vi "Sort.vi"() -> ()   [LabVIEW 2012]
uses:
  <vilib>/Analysis/1siggen.llb/Riffle Array (I32).vi
  <vilib>/Analysis/NI_AALBase.lvlib
panel:
  out "current time":timestamp
  out "Last Max Index":i32
  in  "Reset":bool
  in  "Sort Type:":u16(ring) items=["Labview Sort", "Bubble", "Insertion", "Selection"]
  out "Sort array":i32[](array[numeric])
  in  "EXIT":bool
  in  "GO":bool
  out "Raw Data":waveform(i32)(graph)
  # "There is a 20ms delay in sort loops so that the sorts happen slow enough to veiw.\nThis affects the \"Time took to sort\". Also the sample size is 100 non-recurring numbers from 1-100."
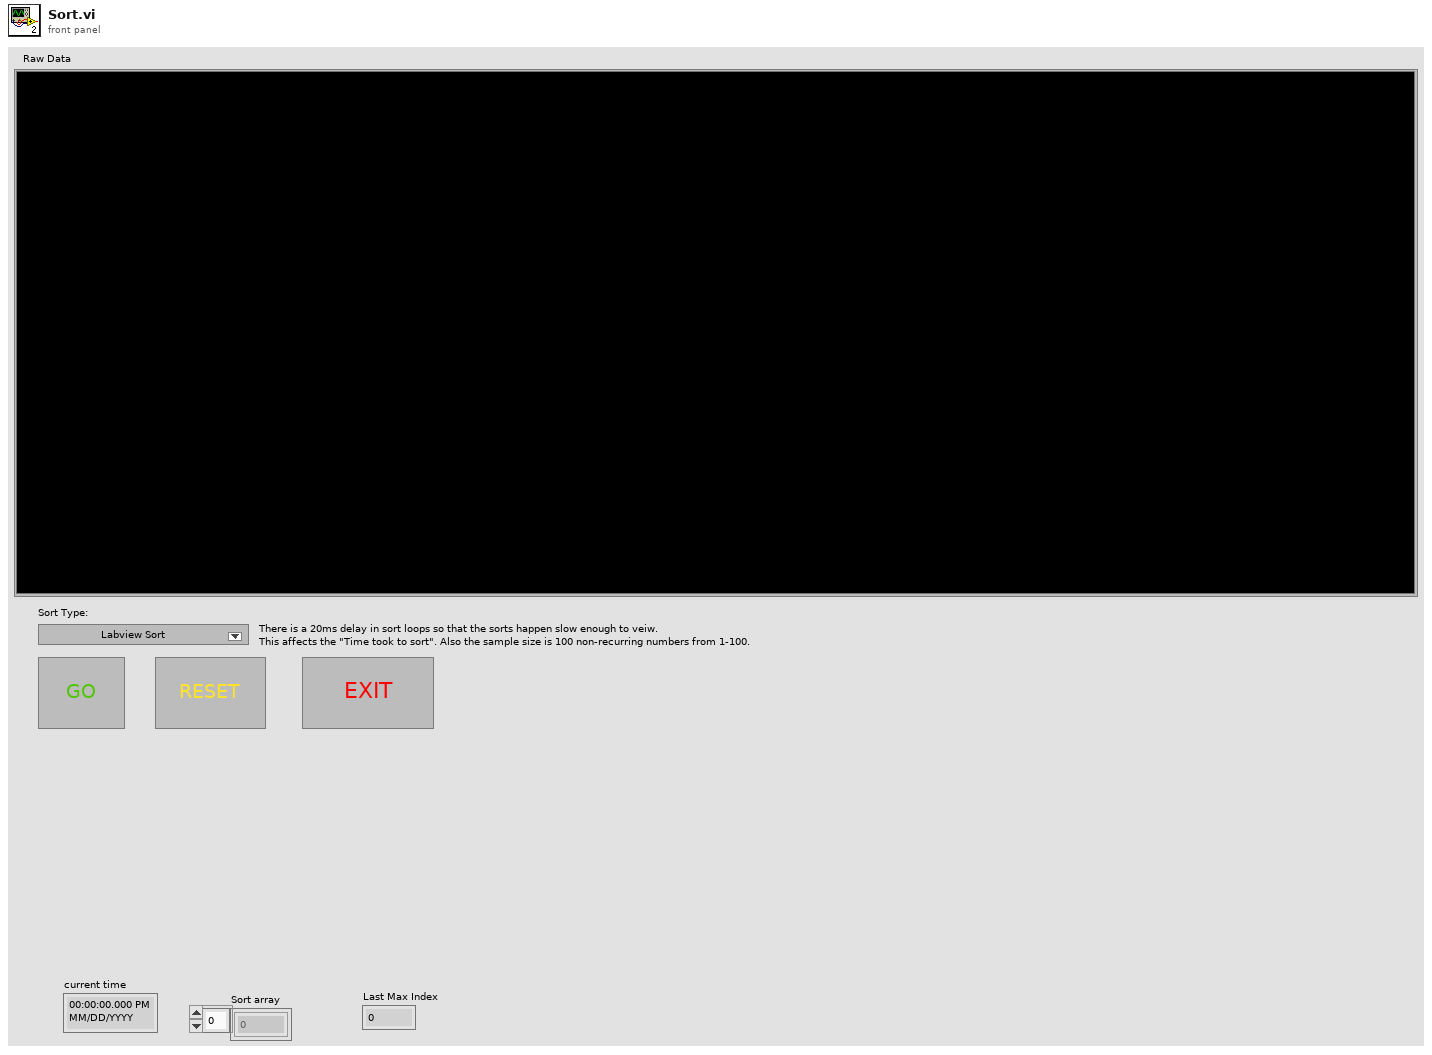
[diagram p1: front panel]
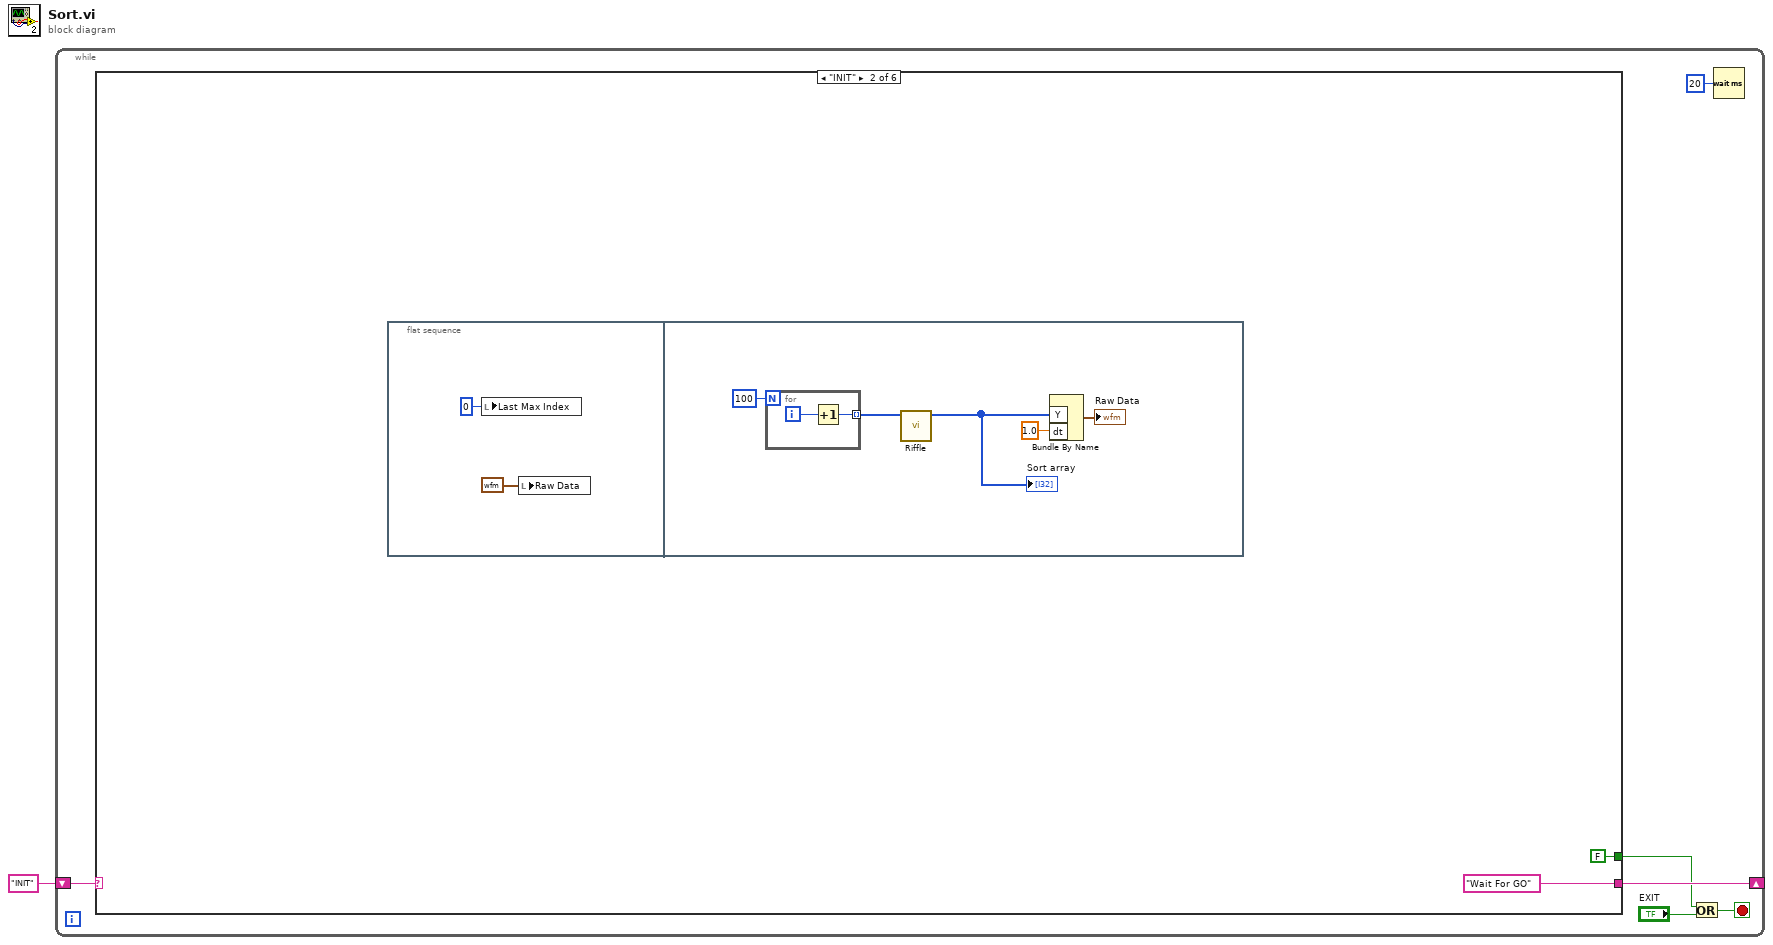
[diagram p0: block diagram]
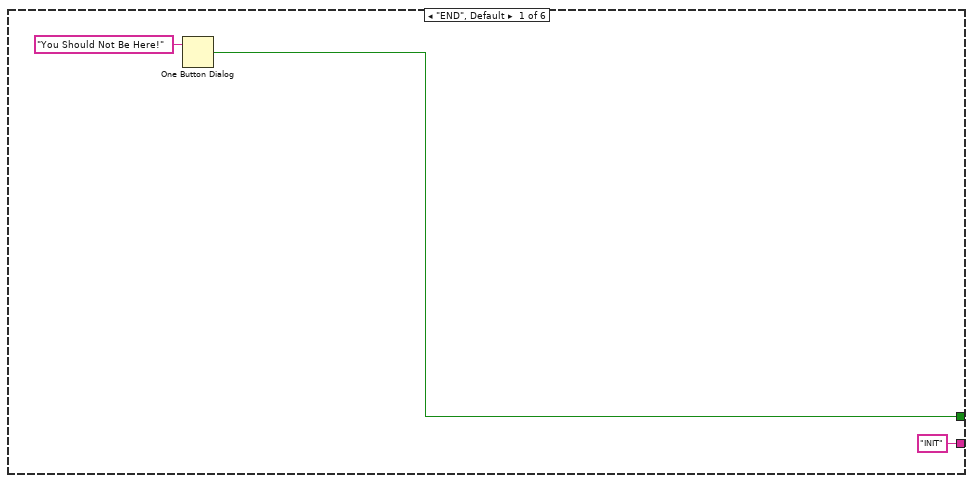
[diagram p2: hidden frame]
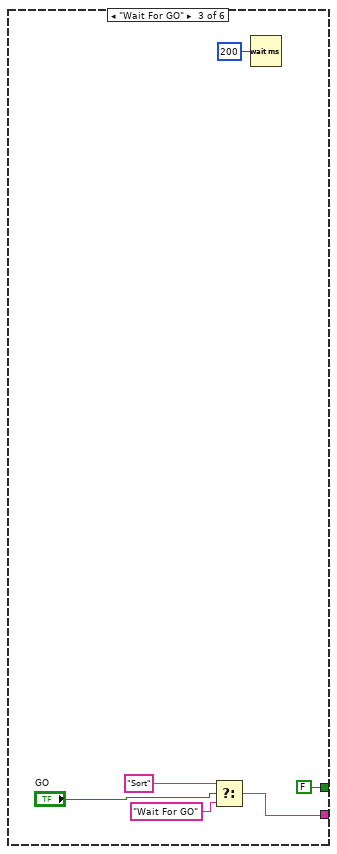
[diagram p3: hidden frame]
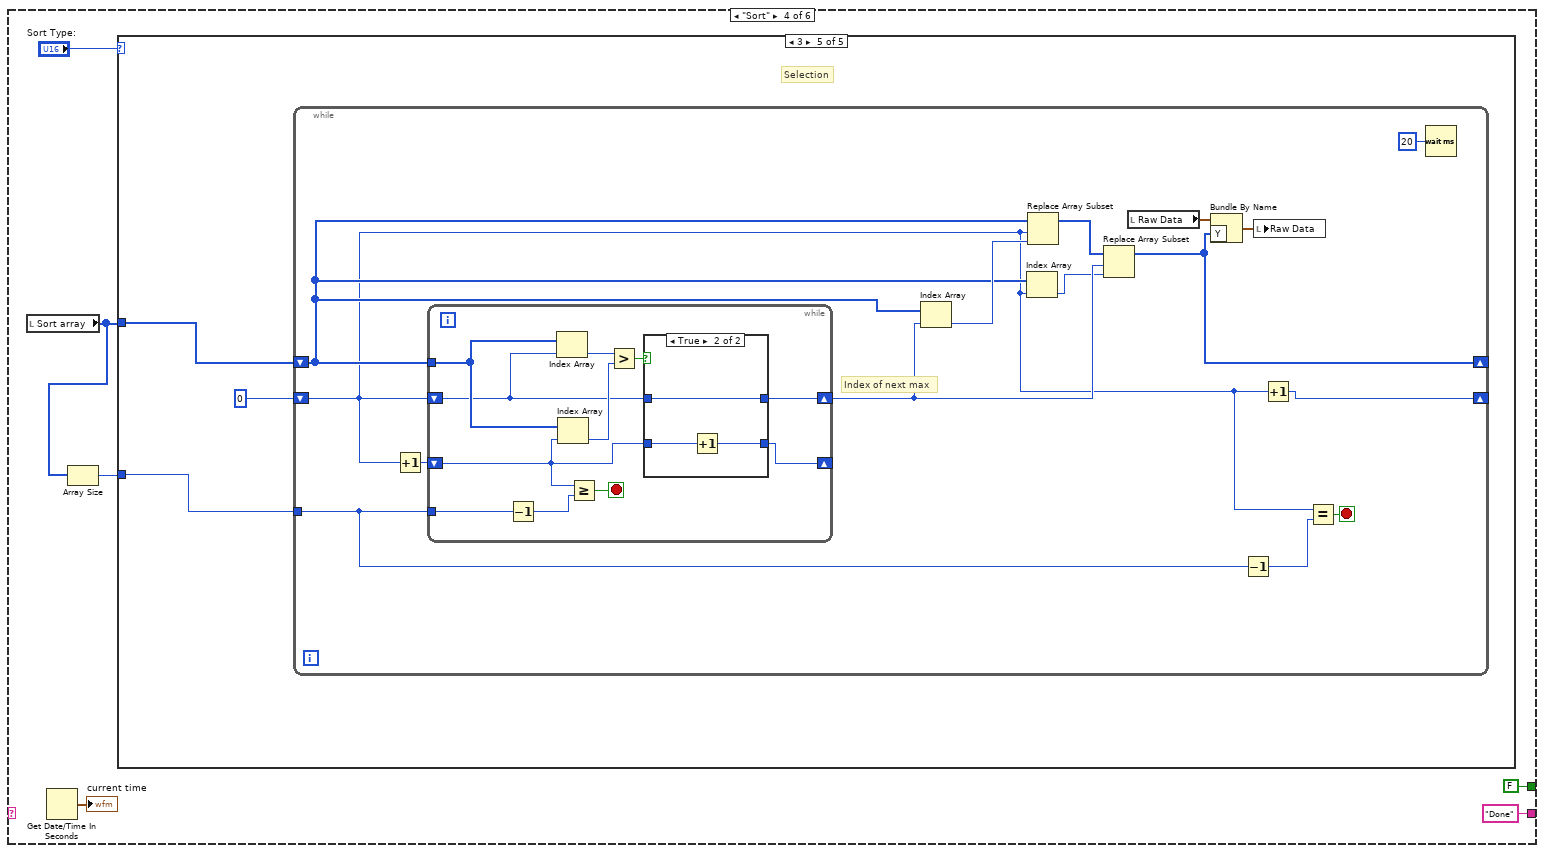
[diagram p4: hidden frame]
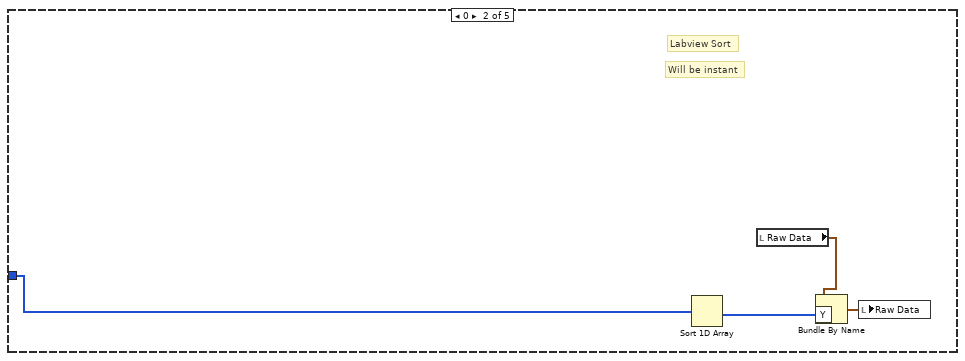
[diagram p6: hidden frame]
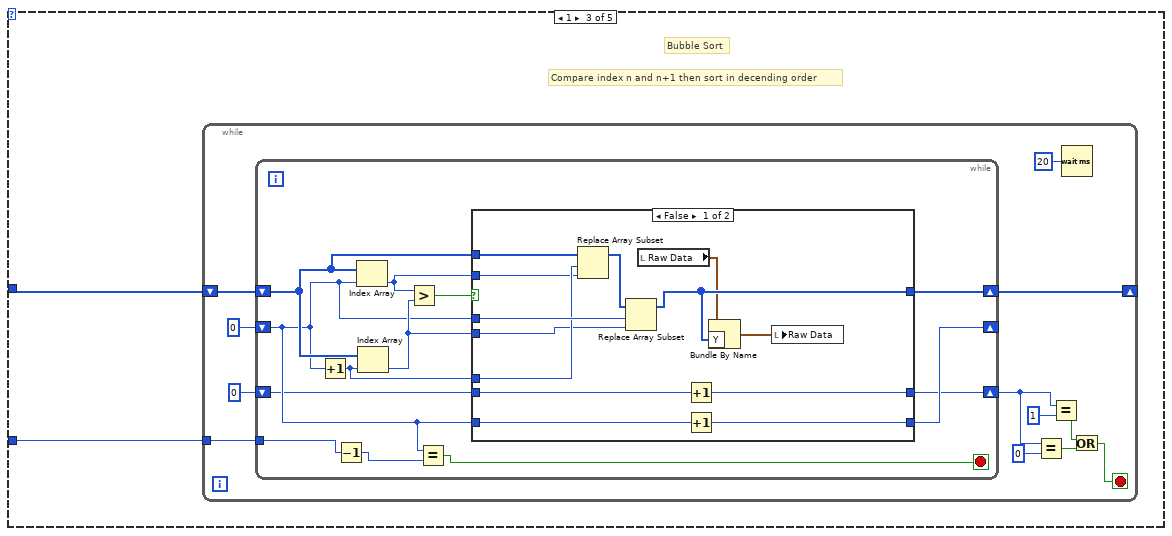
[diagram p7: hidden frame]
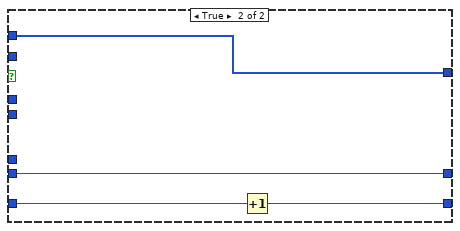
[diagram p8: hidden frame]
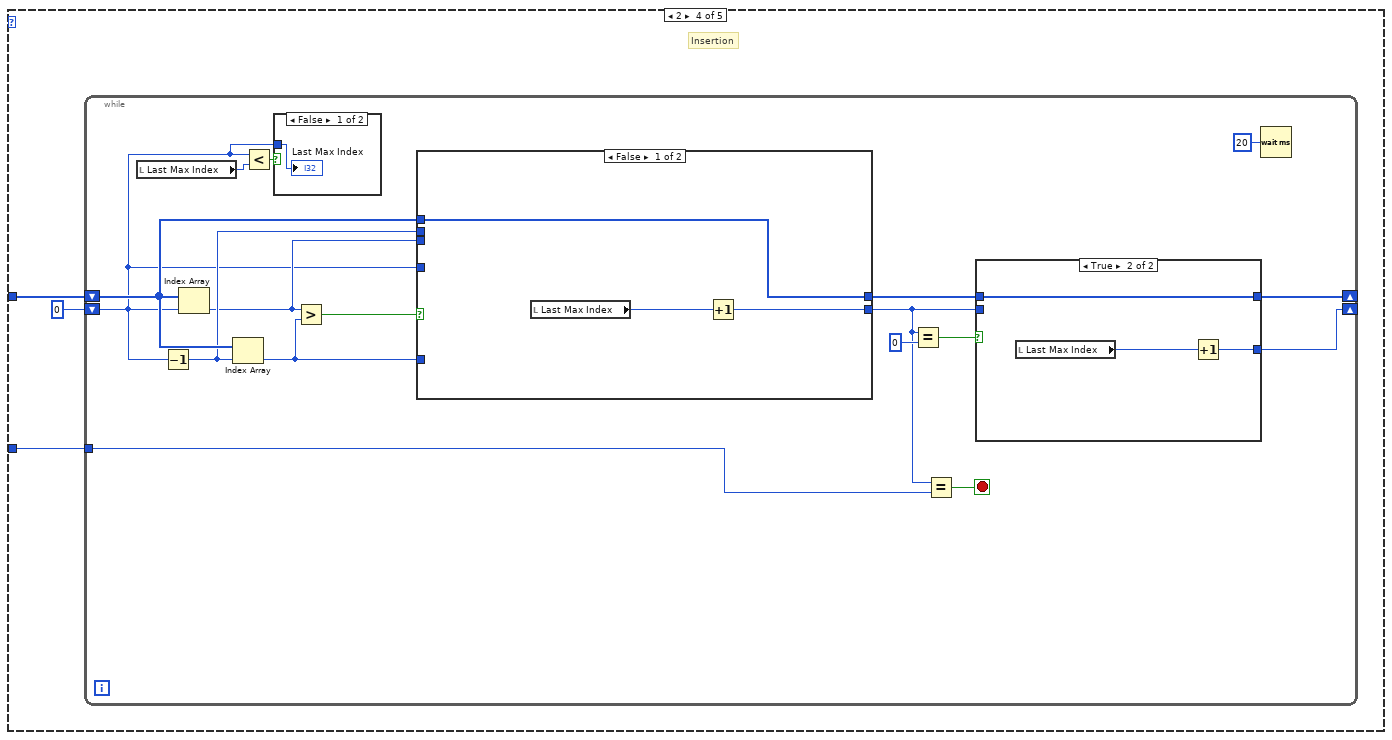
[diagram p9: hidden frame]
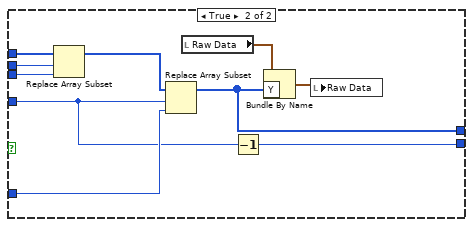
[diagram p12: hidden frame]
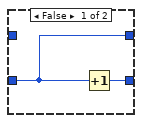
[diagram p13: hidden frame]
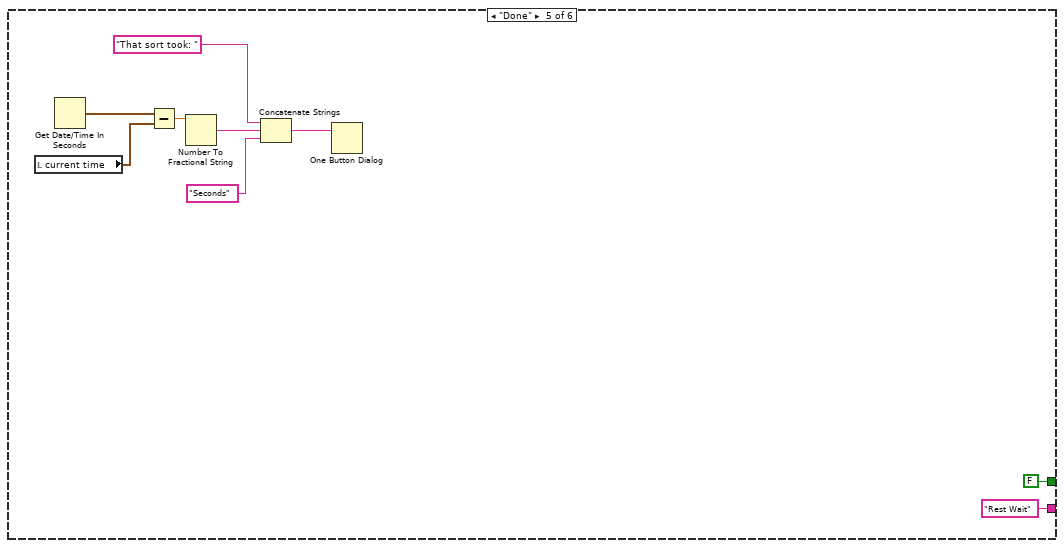
[diagram p14: hidden frame]
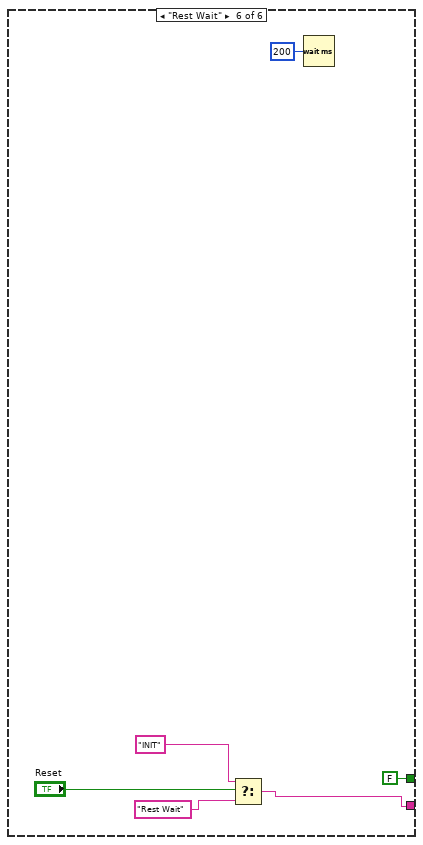
[diagram p15: hidden frame]
diagram:
  n1 = while {
    shift-right: [w5] -> _
    shift-left: "INIT" -> [w6]
    stop <- w4 stop-if-true
    n2 = case shown="\"INIT\"" w6 {
      tunnel: ["INIT" ("f") "Wait For GO" ("f") w23 "Done" ("f") "Rest Wait" ("f") w168] -> w5
      tunnel: [w9 FALSE ("true") FALSE ("true") FALSE ("true") FALSE ("true") FALSE ("true")] -> w2
      frame "END", Default {
        n3 = One Button Dialog(message="You Should Not Be Here!") -> (true=w9:bool)  [unwired: 1 in]
      }
      frame "INIT" {
        n4 = flat-sequence {
          frame #0 {
            n5 = local write "Last Max Index"(0 ("Last Max Index")) -> ()
            n6 = local write "Raw Data"(waveform(dbl) {"t0"=timestamp(0 s since 1904-01-01), "dt"=0.0, "Y"=[]} ("output waveform")) -> ()
          }
          frame #1 {
            n7 = for {
              N: 100 -> [_]
              tunnel: [w20] -> w16 mode=indexing
              i -> [w21]
              n8 = Increment(x=w21) -> (x+1=w20:i32)
            }
            n9 = call-poly <vilib>:"Riffle.vi"("X"=w16) -> ("Riffled {X}"=w15:i32[])  [unwired: 8 in, 2 out]
            "Sort array" <- w15
            n10 = Bundle By Name("Y"=w15, "dt"=1.0) -> (→"Raw Data":waveform(i32))  [unwired: 1 in]
          }
        }
      }
      frame "Wait For GO" {
        n11 = Select(t="Sort", s="GO", f="Wait For GO") -> (s? t:f=w23:string)
        n12 = Wait (ms)(milliseconds to wait=u32 200) -> ()  [unwired: 1 out]
      }
      frame "Sort" {
        n13 = local read "Sort array"() -> (w31:i32[])
        n14 = Get Date/Time In Seconds() -> (seconds since 1Jan1904=→"current time":timestamp)
        n15 = Array Size(array=w31) -> (size(s)=w32:i32)
        n16 = case shown="3" "Sort Type:" {
          tunnel: w32 -> [_ _ w39 w82 w122]
          tunnel: w31 -> [_ w37 w38 w84 w123]
          frame Default {
          }
          frame 0 {
            # "Will be instant"
            # "Labview Sort"
            n17 = Sort 1D Array(array=w37) -> (sorted array=w34:i32[])
            n18 = local read "Raw Data"() -> (w35:waveform(i32))
            n19 = Bundle By Name(cluster=w35, "Y"=w34) -> (w36:waveform(i32))
            n20 = local write "Raw Data"(w36) -> ()
          }
          frame 1 {
            # "Compare index n and n+1 then sort in decending order"
            # "Bubble Sort"
            n21 = while {
              tunnel: w39 -> [w49]
              shift-right: [w48] -> _
              shift-left: w38 -> [w50]
              stop <- w41 stop-if-true
              n22 = while {
                shift-right: [w59] -> w48
                shift-left: w50 -> [w63]
                shift-right: [w58] -> _
                shift-left: 0 ("index (row)") -> [w57]
                tunnel: w49 -> [w56]
                shift-right: [w52] -> w45
                shift-left: 0 ("index (row)") -> [w53]
                stop <- w54 stop-if-true
                n23 = Increment(x=w57) -> (x+1=w62:i32)
                n24 = Decrement(x=w56) -> (x-1=w55:i32)
                n25 = Index Array(array=w63, index=w57) -> (element=w60:i32)
                n26 = Index Array(array=w63, index=w62) -> (element=w61:i32)
                n27 = Greater?(x=w60, y=w61) -> (0:w64:bool)
                n28 = Equal?(x=w57, y=w55) -> (x = y?=w54:bool)
                n29 = case shown="False" w64 {
                  tunnel: w63 -> [w77 w79]
                  tunnel: w57 -> [w76 _]
                  tunnel: w62 -> [w75 _]
                  tunnel: w61 -> [w74 _]
                  tunnel: w60 -> [w73 _]
                  tunnel: [w70 w79] -> w59
                  tunnel: w57 -> [w71 w81]
                  tunnel: [w68 w80] -> w58
                  tunnel: w53 -> [w67 w78]
                  tunnel: [w66 w78] -> w52
                  frame False {
                    n30 = Replace Array Subset(array=w77, new element=w73, index=w75) -> (w72:i32[])
                    n31 = Replace Array Subset(array=w72, new element=w74, index=w76) -> (w70:i32[])
                    n32 = local read "Raw Data"() -> (w65:waveform(i32))
                    n33 = Increment(x=w67) -> (x+1=w66:i32)
                    n34 = Increment(x=w71) -> (x+1=w68:i32)
                    n35 = Bundle By Name(cluster=w65, "Y"=w70) -> (w69:waveform(i32))
                    n36 = local write "Raw Data"(w69) -> ()
                  }
                  frame True {
                    n37 = Increment(x=w81) -> (x+1=w80:i32)
                  }
                }
              }
              n38 = Equal?(x=w45, y=0) -> (x = y?=w43:bool)
              n39 = Equal?(x=w45, y=1) -> (x = y?=w42:bool)
              n40 = Wait (ms)(milliseconds to wait=u32 20) -> ()  [unwired: 1 out]
              n41 = Or(x=w42, y=w43) -> (x .or. y?=w41:bool)
            }
          }
          frame 2 {
            # "Insertion"
            n42 = while {
              shift-right: [w93] -> _
              shift-left: 0 -> [w95]
              shift-right: [w91] -> _
              shift-left: w84 -> [w101]
              tunnel: w82 -> [w86]
              stop <- w88 stop-if-true
              n43 = local read "Last Max Index"() -> (w97:i32)
              n44 = Decrement(x=w95) -> (x-1=w100:i32)
              n45 = Index Array(array=w101, index=w95) -> (element=w99:i32)
              n46 = Index Array(array=w101, index=w100) -> (element=w98:i32)
              n47 = Less?(x=w95, y=w97) -> (x < y?=w96:bool)
              n48 = case shown="False" w96 {
                tunnel: w95 -> [w107 _]
                frame False {
                  "Last Max Index" <- w107
                }
                frame True {
                }
              }
              n49 = Greater?(x=w99, y=w98) -> (0:w89:bool)
              n50 = case shown="False" w89 {
                tunnel: w101 -> [w110 w118]
                tunnel: w100 -> [_ w116]
                tunnel: w99 -> [_ w115]
                tunnel: w95 -> [_ w112]
                tunnel: w98 -> [_ w114]
                tunnel: [w110 w113] -> w92
                tunnel: [w109 w111] -> w87
                frame False {
                  n51 = local read "Last Max Index"() -> (w108:i32)
                  n52 = Increment(x=w108) -> (x+1=w109:i32)
                }
                frame True {
                  n53 = Replace Array Subset(array=w118, new element=w115, index=w116) -> (w117:i32[])
                  n54 = Replace Array Subset(array=w117, new element=w114, index=w112) -> (w113:i32[])
                  n55 = local read "Raw Data"() -> (w120:waveform(i32))
                  n56 = Decrement(x=w112) -> (x-1=w111:i32)
                  n57 = Bundle By Name(cluster=w120, "Y"=w113) -> (w119:waveform(i32))
                  n58 = local write "Raw Data"(w119) -> ()
                }
              }
              n59 = Equal?(x=w87, y=0) -> (x = y?=w90:bool)
              n60 = Equal?(x=w87, y=w86) -> (x = y?=w88:bool)
              n61 = case shown="True" w90 {
                tunnel: [w102 w105] -> w93
                tunnel: w92 -> [w103 w104]
                tunnel: [w103 w104] -> w91
                tunnel: w87 -> [w102 _]
                frame False {
                }
                frame True {
                  n62 = local read "Last Max Index"() -> (w106:i32)
                  n63 = Increment(x=w106) -> (x+1=w105:i32)
                }
              }
              n64 = Wait (ms)(milliseconds to wait=u32 20) -> ()  [unwired: 1 out]
            }
          }
          frame 3 {
            # "Selection"
            n65 = while {
              tunnel: w122 -> [w126]
              shift-right: [w129] -> _
              shift-left: 0 ("index (row)") -> [w125]
              shift-right: [w130] -> _
              shift-left: w123 -> [w132]
              stop <- w128 stop-if-true
              # "Index of next max"
              n66 = Increment(x=w125) -> (x+1=w136:i32)
              n67 = while {
                shift-right: [w143] -> w133
                shift-left: w125 -> [w142]
                tunnel: w126 -> [w146]
                shift-right: [w144] -> _
                shift-left: w136 -> [w141]
                tunnel: w132 -> [w149]
                stop <- w139 stop-if-true
                n68 = Decrement(x=w146) -> (x-1=w140:i32)
                n69 = Index Array(array=w149, index=w142) -> (element=w147:i32)
                n70 = Index Array(array=w149, index=w141) -> (element=w148:i32)
                n71 = Greater Or Equal?(x=w141, y=w140) -> (x >= y?=w139:bool)
                n72 = Greater?(x=w147, y=w148) -> (0:w145:bool)
                n73 = case shown="True" w145 {
                  tunnel: w141 -> [w150 w154]
                  tunnel: [w151 w153] -> w144
                  tunnel: [w150 w152] -> w143
                  tunnel: w142 -> [_ w152]
                  frame False {
                    n74 = Increment(x=w150) -> (x+1=w151:i32)
                  }
                  frame True {
                    n75 = Increment(x=w154) -> (x+1=w153:i32)
                  }
                }
              }
              n76 = Index Array(array=w132, index=w133) -> (element=w135:i32)
              n77 = Index Array(array=w132, index=w125) -> (element=w131:i32)
              n78 = Replace Array Subset(array=w132, new element=w135, index=w125) -> (w134:i32[])
              n79 = Replace Array Subset(array=w134, new element=w131, index=w133) -> (w130:i32[])
              n80 = local read "Raw Data"() -> (w137:waveform(i32))
              n81 = Bundle By Name(cluster=w137, "Y"=w130) -> (w138:waveform(i32))
              n82 = Decrement(x=w126) -> (x-1=w127:i32)
              n83 = local write "Raw Data"(w138) -> ()
              n84 = Increment(x=w125) -> (x+1=w129:i32)
              n85 = Equal?(x=w125, y=w127) -> (x = y?=w128:bool)
              n86 = Wait (ms)(milliseconds to wait=u32 20) -> ()  [unwired: 1 out]
            }
          }
        }
      }
      frame "Done" {
        n87 = local read "current time"() -> (w160:timestamp)
        n88 = Get Date/Time In Seconds() -> (seconds since 1Jan1904=w161:timestamp)
        n89 = Subtract(x=w161, y=w160) -> (x-y=w158:dbl)
        n90 = Number To Fractional String(number=w158) -> (F-format string=w157:string)  [unwired: 3 in]
        n91 = Concatenate Strings("That sort took: " ("message"), w157, "Seconds" ("message")) -> (w156:string)
        n92 = One Button Dialog(message=w156) -> ()  [unwired: 1 in, 1 out]
      }
      frame "Rest Wait" {
        n93 = Select(t="INIT", s="Reset", f="Rest Wait") -> (s? t:f=w168:string)
        n94 = Wait (ms)(milliseconds to wait=u32 200) -> ()  [unwired: 1 out]
      }
    }
    n95 = Or(x=w2, y="EXIT") -> (x .or. y?=w4:bool)
    n96 = Wait (ms)(milliseconds to wait=u32 20) -> ()  [unwired: 1 out]
  }
